vi "Remove Hidden Tags.vi"(8 "error in (no error)":errorcluster, 10 "filenames":string[](array[string]), 11 "Working Dir":path) -> (0 "error out":errorcluster, 3 "Tag Name":string[](array[string]))   [LabVIEW 2024]
uses:
  <userlib>/_OpenG.lib/file/file.llb/openg_file.lvlib
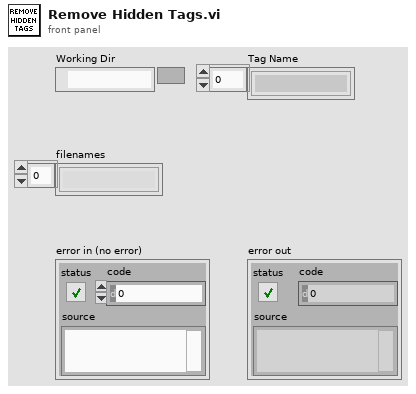
[diagram p1: front panel]
types:
  T1 = typedef "openg_file.lvlib/File Info Record__ogtk.ctl" = cluster{"type":string, "creator":string, "permissions":i32, "data size":i32, "res size":i32, "creation date":u32, "modification date":u32, "bFolder":bool, "bInvisible":bool, "location":cluster{"vertical":i16, "horizontal":i16}, "owner":string, "group":string}
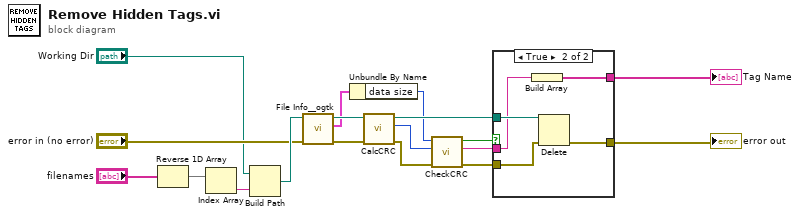
[diagram p0: block diagram]
diagram:
  n1 = Reverse 1D Array(array="filenames") -> (reversed array=w3:string[])
  n2 = Index Array(array=w3) -> (element=w1:string)  [unwired: 1 in]
  n3 = Build Path(base path="Working Dir", name or relative path=w1) -> (appended path=w7:path)
  n4 = call <userlib>:"File Info__ogtk.vi"("error in (no error)"="error in (no error)", "file"=w7) -> ("error out"=w9:errorcluster, "file info"=w6:T1, "file out"=w8:path)  [unwired: 4 in]
  n5 = Unbundle By Name(w6) -> ("data size"=w11:i32)
  n6 = call "CalcCRC.vi"("error in (no error)"=w9, "FileToCalculate"=w8) -> ("error out"=w12:errorcluster, "CRC32Value"=w10:u32, "FileToCalculate out"=w13:path)  [unwired: 7 in]
  n7 = call "CheckCRC.vi"("error in (no error)"=w12, "CRC"=w10, "File Size"=w11) -> ("error out"=w15:errorcluster, "Tag Name"=w17:string, "Found?"=w14:bool)  [unwired: 6 in]
  n8 = case shown="True" w14 {
    tunnel: w13 -> [_ w24]
    tunnel: w15 -> [w19 w23]
    tunnel: [w19 w22] -> w16
    tunnel: w17 -> [_ w21]
    tunnel: [_ w20] -> w18
    frame False {
    }
    frame True {
      n9 = Build Array(w21) -> (w20:string[])
      n10 = Delete(path (use dialog)=w24, error in=w23) -> (error out=w22:errorcluster)  [unwired: 3 in, 2 out]
    }
  }
  "Tag Name" <- w18
  "error out" <- w16
